vi "ABB configure Bearing Inspection.vi"() -> ()   [LabVIEW 2017]
uses:
  ABB global.vi
panel:
  out "Criteria 8":string
  out "Criteria 7":string
  out "Criteria 6":string
  out "Criteria 5":string
  out "Criteria 4":string
  out "Criteria 3":string
  out "Criteria 2":string
  out "Criteria 1":string
  out "Picture 8":picture
  out "Picture 7":picture
  out "Picture 6":picture
  out "Picture 5":picture
  out "Picture 4":picture
  out "Picture 3":picture
  out "Picture 2":picture
  out "Picture 1":picture
  out "Image":picture
  out "Image File":string
  in  "Inspection Category":T1
  in  "Bearing Images":i32(listbox)
  in  "Edit Types":T2
  in  "Exit":bool
  # "Configure Bearing Inspection"
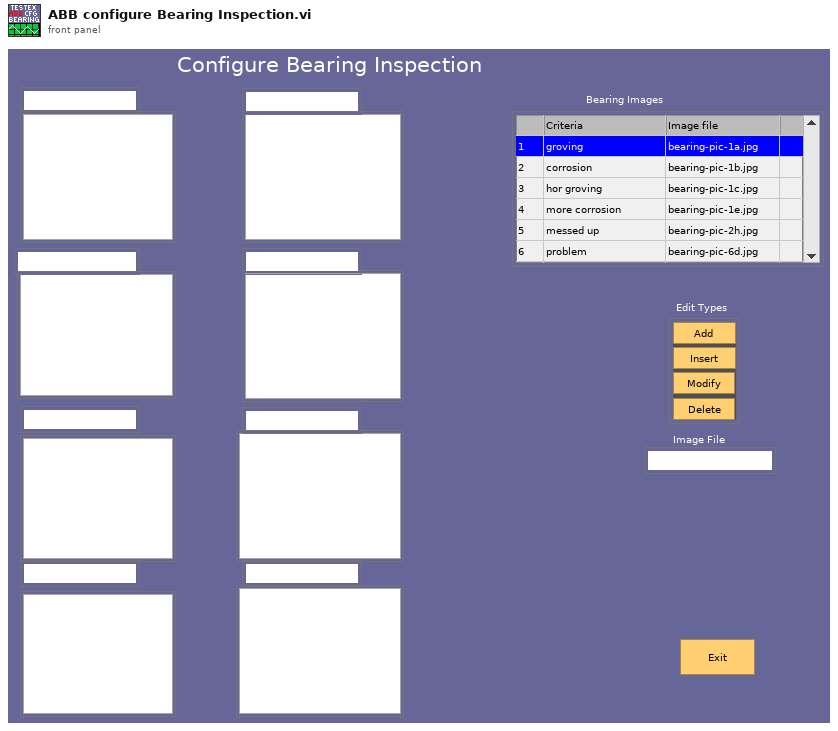
[diagram p1: front panel]
types:
  T1 = cluster{"Criteria":string, "Select Image":bool, "OK":bool, "Cancel":bool}
  T2 = cluster{"Add":bool, "Insert":bool, "Delete":bool, "modify":bool}
  T3 = typedef "imagedata.ctl" = cluster{"image type":i32, "image depth":i32, "image":u8[], "mask":u8[], "colors":u32[], "Rectangle":cluster{"left":i16, "top":i16, "right":i16, "bottom":i16}}
  T4 = enum32{"existing file", "new file", "new or existing file", "existing dir", "new dir", "new or existing dir", "existing file (use LLBs)", "new file (use LLBs)", "new or existing file (use LLBs)", "new or existing file or directory (use LLBs)"}
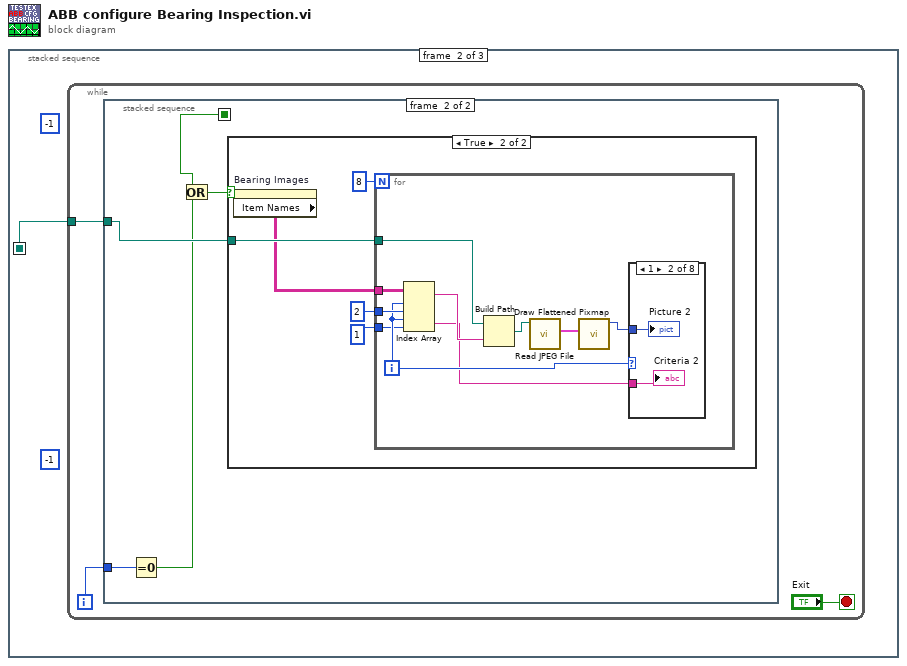
[diagram p0: block diagram]
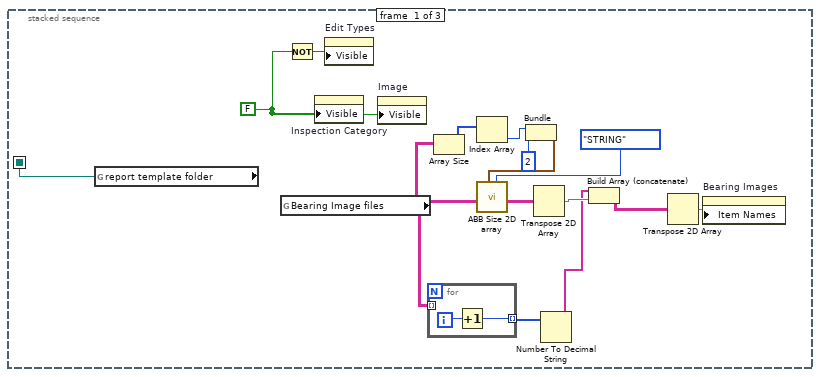
[diagram p2: hidden frame]
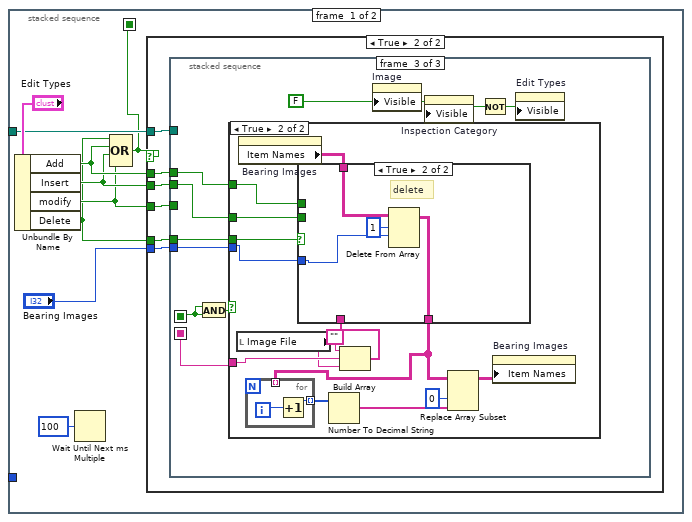
[diagram p3: hidden frame]
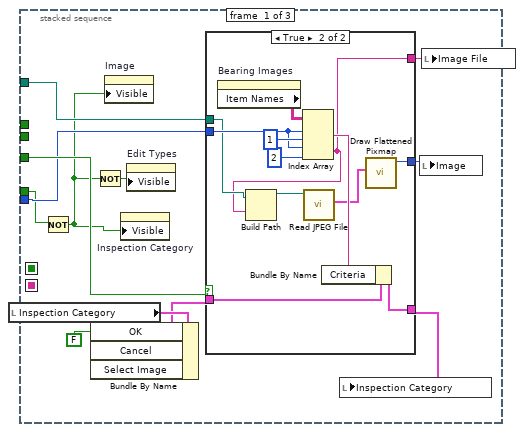
[diagram p5: hidden frame]
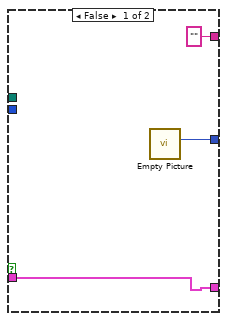
[diagram p6: hidden frame]
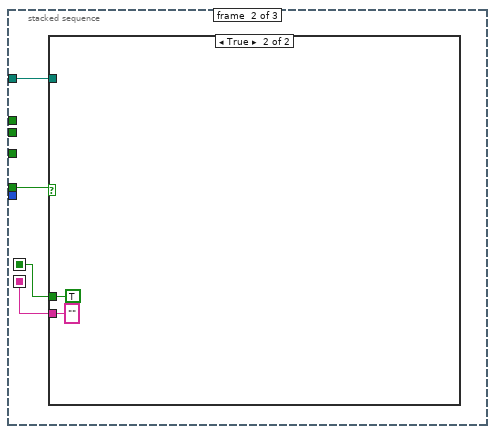
[diagram p7: hidden frame]
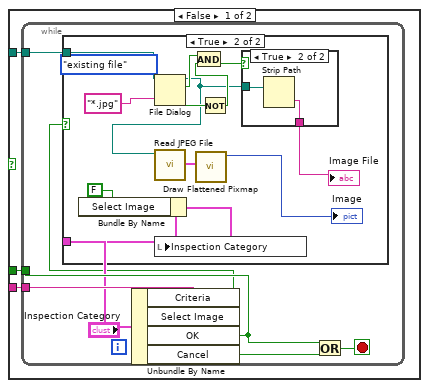
[diagram p8: hidden frame]
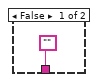
[diagram p10: hidden frame]
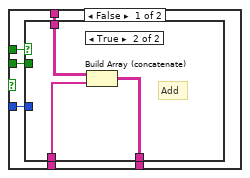
[diagram p12: hidden frame]
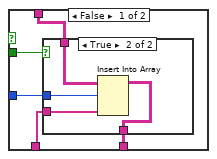
[diagram p13: hidden frame]
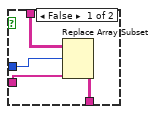
[diagram p14: hidden frame]
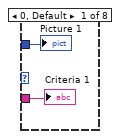
[diagram p16: hidden frame]
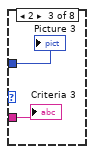
[diagram p17: hidden frame]
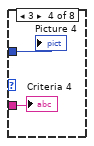
[diagram p18: hidden frame]
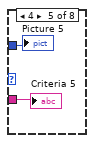
[diagram p19: hidden frame]
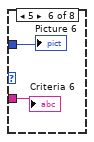
[diagram p20: hidden frame]
diagram:
  n1 = stacked-sequence {
    seq-local: [w14 _ _] -> [_ w18 _]
    frame #0 {
      w7 = FALSE ("Visible")
      n2 = global read "ABB global.vi" "report template folder"() -> (w14:path)
      n3 = global read "ABB global.vi" "Bearing Image files"() -> (w6:string[][])
      n4 = Not(x=w7) -> (.not. x?=w15:bool)
      n5 = property on="Inspection Category" class="Clust (strict)"("Visible"=w7) -> ()  [unwired: 2 in, 2 out]
      n6 = property on="Edit Types" class="Clust"("Visible"=w15) -> ()  [unwired: 2 in, 2 out]
      n7 = property on="Image" class="Pict"("Visible"=w7) -> ()  [unwired: 2 in, 2 out]
      n8 = for {
        tunnel: w6 -> [_] mode=indexing
        tunnel: [w16] -> w5 mode=indexing
        i -> [w17]
        n9 = Increment(x=w17) -> (x+1=w16:i32)
      }
      n10 = Array Size(array=w6) -> (size(s)=w12:i32[])
      n11 = Index Array(array=w12) -> (element=w11:i32)  [unwired: 1 in]
      n12 = Bundle(w11, 2) -> (w9:cluster{i32, i32})  [unwired: 1 in]
      n13 = call "ABB Size 2D array.vi"("Type"=enum16{"Integer", "DBL", "STRING", "BOOLEAN"}."STRING", "Size"=w9, "String Array in"=w6) -> ("String Array out"=w13:string[][])  [unwired: 5 in, 3 out]
      n14 = Transpose 2D Array(2D array=w13) -> (transposed array=w4:string[][])
      n15 = Number To Decimal String(number=w5) -> (decimal integer string=w2:string[])  [unwired: 1 in]
      n16 = Build Array (concatenate)(w2, w4) -> (w3:string[][])
      n17 = Transpose 2D Array(2D array=w3) -> (transposed array=w1:string[][])
      n18 = property on="Bearing Images" class="MCListbox (strict)"("Item Names"=w1) -> ()  [unwired: 2 in, 2 out]
    }
    frame #1 {
      (unwired) -1 ("Noise Test Images")
      (unwired) -1 ("Number Values")
      n19 = while {
        tunnel: w18 -> [w20]
        i -> [w19]
        stop <- "Exit" stop-if-true
        n20 = stacked-sequence {
          seq-local: [w22 _] -> [_ w150]
          tunnel: w20 -> [w28 w151]
          tunnel: w19 -> [_ w149]
          frame #0 {
            n21 = Unbundle By Name("Edit Types") -> ("Add"=w27:bool, "Insert"=w26:bool, "modify"=w24:bool, "Delete"=w23:bool)
            n22 = Wait Until Next ms Multiple(millisecond multiple=u32 100) -> ()  [unwired: 1 out]
            n23 = Compound Arithmetic op=OR(w23, w27, w26, w24) -> (w22:bool)
            n24 = case shown="True" w22 {
              tunnel: w28 -> [_ w36]
              tunnel: "Bearing Images" -> [_ w35]
              tunnel: w27 -> [_ w34]
              tunnel: w26 -> [_ w33]
              tunnel: w24 -> [_ w32]
              tunnel: w23 -> [_ w31]
              frame False {
              }
              frame True {
                n25 = stacked-sequence {
                  seq-local: [_ w67 _] -> [_ _ w98]
                  seq-local: [_ w65 _] -> [_ _ w104]
                  tunnel: w36 -> [w40 w66 _]
                  tunnel: w35 -> [w46 _ w103]
                  tunnel: w34 -> [_ _ w102]
                  tunnel: w33 -> [_ _ w101]
                  tunnel: w32 -> [w47 _ _]
                  tunnel: w31 -> [w38 w64 w96]
                  frame #0 {
                    w42 = FALSE
                    n26 = local read "Inspection Category"() -> (w44:T1)
                    n27 = Not(x=w38) -> (.not. x?=w37:bool)
                    n28 = Bundle By Name(cluster=w44, "OK"=w42, "Cancel"=w42, "Select Image"=w42) -> (w43:T1)
                    n29 = Not(x=w37) -> (.not. x?=w48:bool)
                    n30 = property on="Image" class="Pict"("Visible"=w37) -> ()  [unwired: 2 in, 2 out]
                    n31 = property on="Inspection Category" class="Clust (strict)"("Visible"=w37) -> ()  [unwired: 2 in, 2 out]
                    n32 = property on="Edit Types" class="Clust"("Visible"=w48) -> ()  [unwired: 2 in, 2 out]
                    n33 = case shown="True" w47 {
                      tunnel: w46 -> [_ w57]
                      tunnel: w43 -> [w51 w59]
                      tunnel: [w51 w58] -> w45
                      tunnel: [w50 w55] -> w41
                      tunnel: w40 -> [_ w54]
                      tunnel: ["" w52] -> w39
                      frame False {
                        n34 = call "Empty Picture"() -> ("empty picture"=w50:picture)
                      }
                      frame True {
                        n35 = property on="Bearing Images" class="MCListbox (strict)"() -> ("Item Names"=w63:string[][])  [unwired: 2 in, 2 out]
                        n36 = Index Array(array=w63, index (row) #1=w57, index (col) #1=1 ("disabled index (col)"), index (row) #2=w57, index (col) #2=2 ("disabled index (col)")) -> (element #1=w60:string, element #2=w52:string)
                        n37 = Build Path(base path=w54, name or relative path=w52) -> (appended path=w53:path)
                        n38 = call <vilib>:"Read JPEG File.vi"("path to JPEG file"=w53) -> ("image data"=w56:T3)  [unwired: 8 in, 2 out]
                        n39 = Bundle By Name(cluster=w59, "Criteria"=w60) -> (w58:T1)
                        n40 = call <vilib>:"Draw Flattened Pixmap.vi"("image data"=w56) -> ("new picture"=w55:picture)  [unwired: 8 in]
                      }
                    }
                    n41 = local write "Inspection Category"(w45) -> ()
                    n42 = local write "Image"(w41) -> ()
                    n43 = local write "Image File"(w39) -> ()
                  }
                  frame #1 {
                    n44 = case shown="True" w64 {
                      tunnel: [w70 TRUE ("OK")] -> w67
                      tunnel: w66 -> [w69 _]
                      tunnel: [w68 "" ("Criteria")] -> w65
                      frame False {
                        n45 = while {
                          tunnel: [w75] -> w70
                          tunnel: w69 -> [w74]
                          tunnel: [w73] -> w68
                          stop <- w76 stop-if-true
                          n46 = Unbundle By Name("Inspection Category") -> ("Criteria"=w73:string, "Select Image"=w71:bool, "OK"=w75:bool, "Cancel"=w77:bool)
                          n47 = case shown="True" w71 {
                            tunnel: w74 -> [_ w89]
                            tunnel: "Inspection Category" -> [_ w81]
                            frame False {
                            }
                            frame True {
                              (unwired) T4."existing file" ("select mode (2)")
                              n48 = Bundle By Name(cluster=w81, "Select Image"=FALSE) -> (w80:T1)
                              n49 = File Dialog(6:"*.jpg" ("pattern"), 11:w89) -> (1:w87:bool, 2:w88:bool, 3:w83:path)  [unwired: 5 in, 1 out]
                              n50 = call <vilib>:"Read JPEG File.vi"("path to JPEG file"=w83) -> ("image data"=w82:T3)  [unwired: 8 in, 2 out]
                              n51 = local write "Inspection Category"(w80) -> ()
                              n52 = call <vilib>:"Draw Flattened Pixmap.vi"("image data"=w82) -> ("new picture"=→"Image":picture)  [unwired: 8 in]
                              n53 = Not(x=w87) -> (.not. x?=w86:bool)
                              n54 = And(x=w88, y=w86) -> (x .and. y?=w84:bool)
                              n55 = case shown="True" w84 {
                                tunnel: w83 -> [_ w93]
                                tunnel: ["" w92] -> w85
                                frame False {
                                }
                                frame True {
                                n56 = Strip Path(path=w93) -> (name=w92:string)  [unwired: 1 out]
                                }
                              }
                              "Image File" <- w85
                            }
                          }
                          n57 = Or(x=w75, y=w77) -> (x .or. y?=w76:bool)
                        }
                      }
                      frame True {
                      }
                    }
                  }
                  frame #2 {
                    w97 = FALSE ("Visible")
                    n58 = And(x=w98, y=w98) -> (x .and. y?=w100:bool)
                    n59 = case shown="True" w100 {
                      tunnel: w104 -> [_ w116]
                      tunnel: w103 -> [_ w112]
                      tunnel: w102 -> [_ w118]
                      tunnel: w101 -> [_ w113]
                      tunnel: w96 -> [_ w105]
                      frame False {
                      }
                      frame True {
                        n60 = local read "Image File"() -> (w115:string)
                        n61 = property on="Bearing Images" class="MCListbox (strict)"() -> ("Item Names"=w117:string[][])  [unwired: 2 in, 2 out]
                        n62 = Build Array("", w116, w115) -> (w114:string[])
                        n63 = case shown="True" w105 {
                          tunnel: w118 -> [w124 _]
                          tunnel: w117 -> [w123 w144]
                          tunnel: w114 -> [w122 _]
                          tunnel: w113 -> [w121 _]
                          tunnel: w112 -> [w120 w142]
                          tunnel: [w119 w141] -> w109
                          frame False {
                            n64 = case shown="True" w124 {
                              tunnel: w123 -> [w128 w140]
                              tunnel: [w126 w138] -> w119
                              tunnel: w122 -> [w125 w139]
                              tunnel: w121 -> [w129 _]
                              tunnel: w120 -> [w127 _]
                              frame False {
                                n65 = case shown="True" w129 {
                                tunnel: w128 -> [w133 w137]
                                tunnel: w127 -> [w132 w136]
                                tunnel: [w130 w135] -> w126
                                tunnel: w125 -> [w131 w134]
                                frame False {
                                n66 = Replace Array Subset "Replace Array Subset"(array=w133, new element=w131, index (row)=w132) -> (w130:string[][])  [unwired: 1 in]
                                }
                                frame True {
                                n67 = Insert Into Array "Insert Into Array"(array=w137, index (row)=w136, new element=w134) -> (w135:string[][])  [unwired: 1 in]
                                }
                                }
                              }
                              frame True {
                                # "Add"
                                n68 = Build Array (concatenate)(w140, w139) -> (w138:string[][])
                              }
                            }
                          }
                          frame True {
                            # "delete"
                            n69 = Delete From Array(array=w144, length=1, index (row)=w142) -> (array with subset deleted=w141:string[][])  [unwired: 1 in, 1 out]
                          }
                        }
                        n70 = for {
                          tunnel: w109 -> [_] mode=indexing
                          tunnel: [w145] -> w110 mode=indexing
                          i -> [w146]
                          n71 = Increment(x=w146) -> (x+1=w145:i32)
                        }
                        n72 = Number To Decimal String(number=w110) -> (decimal integer string=w107:string[])  [unwired: 1 in]
                        n73 = Replace Array Subset(array=w109, new element=w107, index (col)=0 ("disabled index (col)")) -> (w106:string[][])  [unwired: 1 in]
                        n74 = property on="Bearing Images" class="MCListbox (strict)"("Item Names"=w106) -> ()  [unwired: 2 in, 2 out]
                      }
                    }
                    n75 = property on="Image" class="Pict"("Visible"=w97) -> ()  [unwired: 2 in, 2 out]
                    n76 = property on="Inspection Category" class="Clust (strict)"("Visible"=w97) -> ()  [unwired: 2 in, 2 out]
                    n77 = Not(x=w97) -> (.not. x?=w99:bool)
                    n78 = property on="Edit Types" class="Clust"("Visible"=w99) -> ()  [unwired: 2 in, 2 out]
                  }
                }
              }
            }
          }
          frame #1 {
            n79 = Equal To 0?(x=w149) -> (x = 0?=w148:bool)
            n80 = Or(x=w150, y=w148) -> (x .or. y?=w147:bool)
            n81 = case shown="True" w147 {
              tunnel: w151 -> [_ w155]
              frame False {
              }
              frame True {
                n82 = property on="Bearing Images" class="MCListbox (strict)"() -> ("Item Names"=w154:string[][])  [unwired: 2 in, 2 out]
                n83 = for {
                  N: 8 -> [_]
                  tunnel: w154 -> [w166]
                  tunnel: 2 ("disabled index (col)") -> [w160]
                  tunnel: w155 -> [w161]
                  tunnel: 1 ("disabled index (col)") -> [w158]
                  i -> [w159]
                  n84 = Index Array(array=w166, index (row) #1=w159, index (col) #1=w160, index (row) #2=w159, index (col) #2=w158) -> (element #1=w162:string, element #2=w157:string)
                  n85 = Build Path(base path=w161, name or relative path=w162) -> (appended path=w164:path)
                  n86 = call <vilib>:"Read JPEG File.vi"("path to JPEG file"=w164) -> ("image data"=w165:T3)  [unwired: 8 in, 2 out]
                  n87 = call <vilib>:"Draw Flattened Pixmap.vi"("image data"=w165) -> ("new picture"=w163:picture)  [unwired: 8 in]
                  n88 = case shown="1" w159 {
                    tunnel: w163 -> [w168 w169 w172 w174 w176 w178 w180 w181]
                    tunnel: w157 -> [w167 w170 w171 w173 w175 w177 w179 w182]
                    frame 0, Default {
                      "Picture 1" <- w168
                      "Criteria 1" <- w167
                    }
                    frame 1 {
                      "Picture 2" <- w169
                      "Criteria 2" <- w170
                    }
                    frame 2 {
                      "Criteria 3" <- w171
                      "Picture 3" <- w172
                    }
                    frame 3 {
                      "Picture 4" <- w174
                      "Criteria 4" <- w173
                    }
                    frame 4 {
                      "Picture 5" <- w176
                      "Criteria 5" <- w175
                    }
                    frame 5 {
                      "Picture 6" <- w178
                      "Criteria 6" <- w177
                    }
                    frame 6 {
                      "Picture 7" <- w180
                      "Criteria 7" <- w179
                    }
                    frame 7 {
                      "Picture 8" <- w181
                      "Criteria 8" <- w182
                    }
                  }
                }
              }
            }
          }
        }
      }
    }
    frame #2 {
      n89 = Two Button Dialog(message="Save any Changes?") -> (T button?=w184:bool)  [unwired: 2 in]
      n90 = case shown="True" w184 {
        frame False {
        }
        frame True {
          n91 = stacked-sequence {
            frame #0 {
              n92 = property on="Bearing Images" class="MCListbox (strict)"() -> ("Item Names"=w188:string[][])  [unwired: 2 in, 2 out]
              n93 = Array Subset(array=w188, index (col)=1 ("index"), length (col)=2 ("length")) -> (w186:string[][])  [unwired: 2 in]
              n94 = global write "ABB global.vi" "Bearing Image files"(w186) -> ()
            }
            frame #1 {
              n95 = call "ABB Load-Save config.vi"("confirm save"=FALSE, "Mode"=enum16{"LOAD", "SAVE"}."SAVE") -> ()  [unwired: 10 in]
            }
          }
        }
      }
    }
  }
